vi "StateSpaceTest.vi"() -> ()   [LabVIEW 2017]
uses:
  <vilib>/Analysis/Matrix/Datatypes/RealMatrix.ctl
  <vilib>/Analysis/Matrix/Datatypes/ComplexMatrix.ctl
  <vilib>/Analysis/Matrix/NI_Matrix.lvlib
panel:
  in  "Poles":T1=[[-5.0+0.0i], [-10.0+0.0i]]
  in  "goal_next":T2=[[8.0], [0.0]]
  out "Waveform Chart":cluster{"Real Matrix Element":dbl, "y":dbl}(graph)={"Real Matrix Element"=8.0, "y"=7.999993730241449}
  in  "Plant":T3={"Gains"={"A"=[[0.0, 1.0], [0.0, -1.0]], "B"=[[0.0], [1.0]], "C"=[[1.0, 0.0]], "D"=[[0.0]], "Q"=[], "R"=[], "K"=[], "Kff"=[], "L"=[]}, "X"=[[0.0], [0.0]]}
  in  "u":dbl(slide)=-0.00012336390241478301 scale=-12.0..12.0
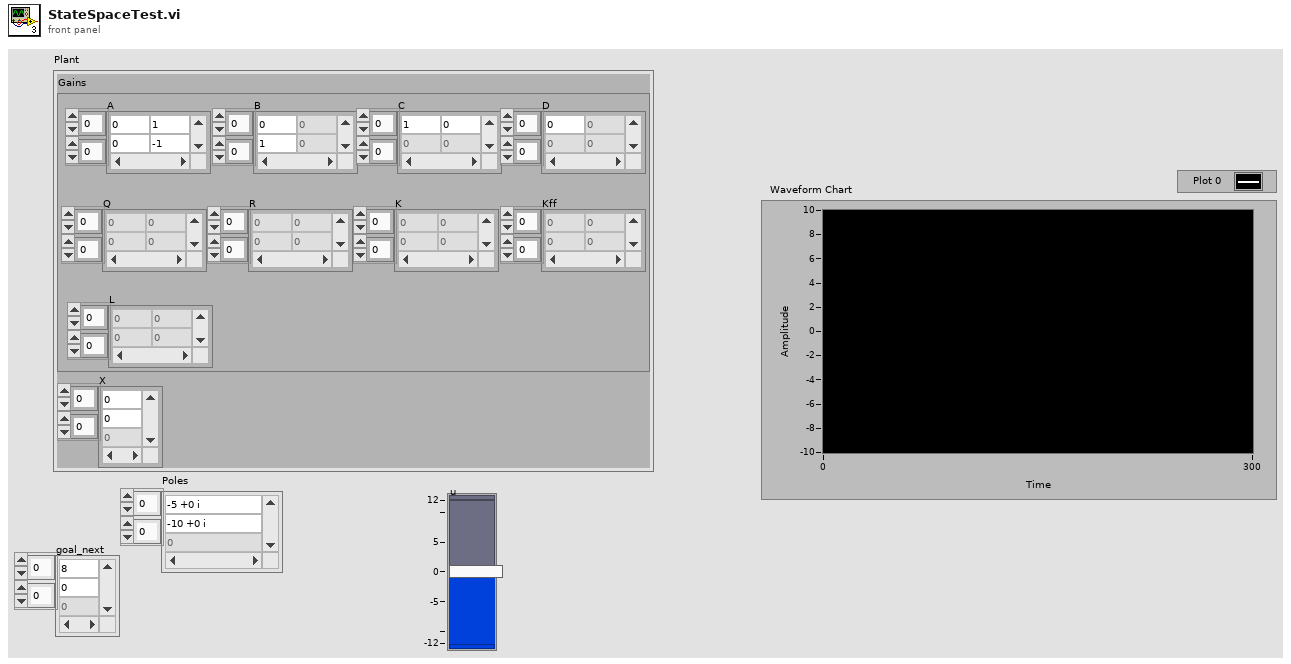
[diagram p1: front panel]
types:
  T1 = typedef "NI_Matrix.lvlib/ComplexMatrix.ctl" = cdb[][]
  T2 = typedef "NI_Matrix.lvlib/RealMatrix.ctl" = dbl[][]
  T3 = cluster{"Gains":cluster{"A":T2, "B":T2, "C":T2, "D":T2, "Q":T2, "R":T2, "K":T2, "Kff":T2, "L":T2}, "X":T2}
  T4 = cluster{"A":T2, "B":T2, "C":T2, "D":T2, "Q":T2, "R":T2, "K":T2, "Kff":T2, "L":T2}
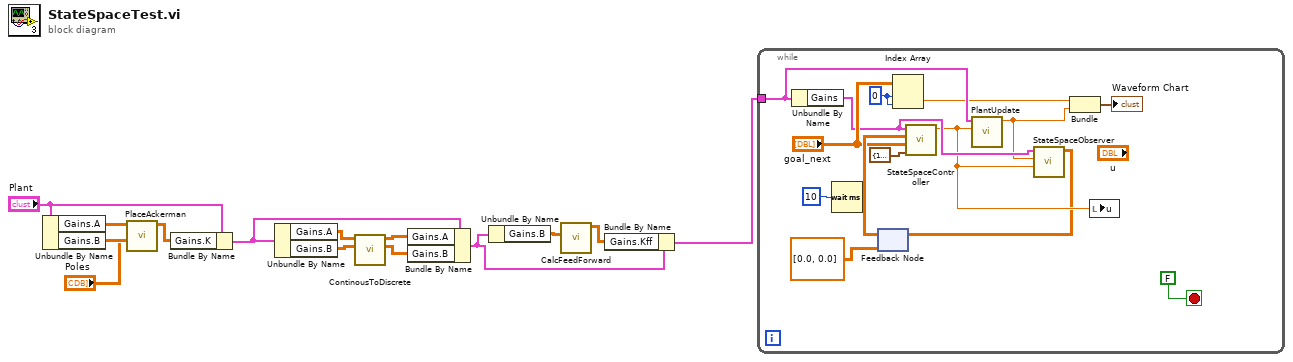
[diagram p0: block diagram]
diagram:
  n1 = Unbundle By Name("Plant") -> ("Gains.A"=w6:T2, "Gains.B"=w5:T2)
  n2 = call "PlaceAckerman.vi"("Poles"="Poles", "B"=w5, "A"=w6) -> ("K"=w2:T2)  [unwired: 8 in]
  n3 = Bundle By Name(cluster="Plant", "Gains.K"=w2) -> (w1:T3)
  n4 = Unbundle By Name(w1) -> ("Gains.A"=w14:T2, "Gains.B"=w13:T2)
  n5 = call "ContinousToDiscrete.vi"("B"=w13, "A"=w14) -> ("B_d"=w11:T2, "A_d"=w12:T2)  [unwired: 8 in]
  n6 = Bundle By Name(cluster=w1, "Gains.A"=w12, "Gains.B"=w11) -> (w9:T3)
  n7 = Unbundle By Name(w9) -> ("Gains.B"=w10:T2)
  n8 = call "CalcFeedForward.vi"("B"=w10) -> ("Kff"=w7:T2)  [unwired: 10 in]
  n9 = Bundle By Name(cluster=w9, "Gains.Kff"=w7) -> (w8:T3)
  n10 = while {
    tunnel: w8 -> [w25]
    stop <- FALSE stop-if-true
    w21 = 0 ("index (row)")
    n11 = Unbundle By Name(w25) -> ("Gains"=w18:T4)
    n12 = Wait (ms)(milliseconds to wait=u32 10) -> ()  [unwired: 1 out]
    n13 = feedback #1(T2 [[0.0], [0.0]] ("X")) -> (w24:T2)
    n14 = Index Array(array="goal_next", index (row)=w21, index (col)=w21) -> (element=w20:dbl)
    n15 = call "StateSpaceController.vi"("u_Range"=cluster{"u_max":dbl, "u_min":dbl} {"u_max"=12.0, "u_min"=-12.0}, "goal_next"="goal_next", "x"=w24, "Gains"=w18) -> ("u"=w16:dbl)  [unwired: 7 in]
    n16 = call "PlantUpdate.vi"("u"=w16, "Plant"=w25) -> ("y"=w17:dbl)  [unwired: 8 in, 1 out]
    n17 = call "StateSpaceObserver.vi"("u"=w16, "y"=w17, "Gains"=w18) -> ("X_hat"=w15:T2)  [unwired: 8 in]
    n18 = feedback-in #1(w15) -> ()
    n19 = Bundle("Real Matrix Element"=w20, "y"=w17) -> (→"Waveform Chart":cluster{"Real Matrix Element":dbl, "y":dbl})  [unwired: 1 in]
    n20 = local write "u"(w16) -> ()
  }
